vi "Attempt to Start Controller.vi"(8 "error in (no error)":errorcluster, 11 "Test Step Controller in":refnum<class "Server Controller.lvclass">) -> (0 "error out":errorcluster)   [LabVIEW 2026, in "Server Controller.lvlib" / "Server Controller.lvclass"]
uses:
  Server Controller.lvclass
  Server Controller.lvclass/Server Controller.ctl
  MAL-Framework/user.lib/Common Components/Controller/Controller.lvclass
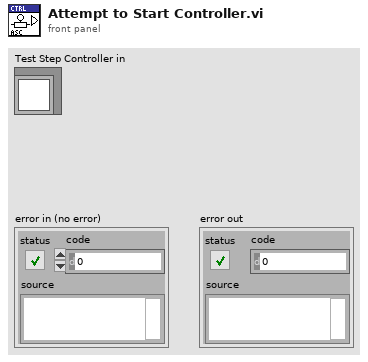
[diagram p1: front panel]
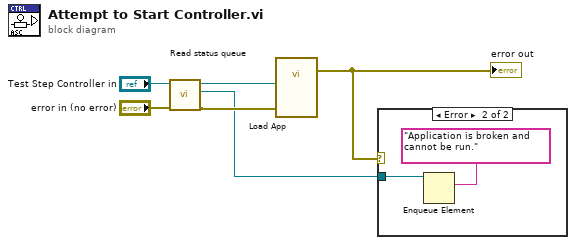
[diagram p0: block diagram]
diagram:
  n1 = call "Read status queue.vi"("error in (no error)"="error in (no error)", "Controller in"="Test Step Controller in") -> ("error out"=w3:errorcluster, "status queue"=w2:refnum<queue>, "Controller out"=w1:refnum<class "Server Controller.lvclass">)  [unwired: 7 in]
  n2 = call-by-ref "Load App.vi"("error in (no error)"=w3, "Controller Actor.lvlib:Controller.lvclass"=w1) -> (error out=w6:errorcluster)  [unwired: 11 in, 2 out]
  "error out" <- w6
  n3 = case shown="Error" w6 {
    tunnel: w2 -> [_ w7]
    frame No Error {
    }
    frame Error {
      n4 = Enqueue Element(queue=w7, element="Application is broken and cannot be run." ("notification")) -> ()  [unwired: 2 in, 3 out]
    }
  }
